vi "SetPosition.vi"(7 "AltPipe?":bool, 8 "error in (no error)":errorcluster, 9 "Position":T1=enum."C0, Cargo Ground", 10 "Hatch Grabbed?":bool, 11 "Elevator Concrete in":refnum<class "Elevator Linear.lvclass">) -> (0 "error out":errorcluster, 3 "Elevator Concrete out":refnum<class "Elevator Linear.lvclass">)   [LabVIEW 2018, in "Elevator.lvlib" / "Elevator Linear.lvclass"]
uses:
  Elevator Linear.lvclass
  C:/Users/Public/Documents/2019DeepSpace/Classes/Elevator/Elevator.lvclass
  Controls/Elevator Position.ctl
  Elevator Linear.lvclass/Elevator Linear.ctl
  Elevator.lvclass/Elevator.ctl
  Public Methods/Read Arm Position Values.vi
  <vilib>/Rock Robotics/Network Tables/NT Write Number.vi
  <vilib>/Rock Robotics/Network Tables/NT Write String.vi
  Elevator.lvclass
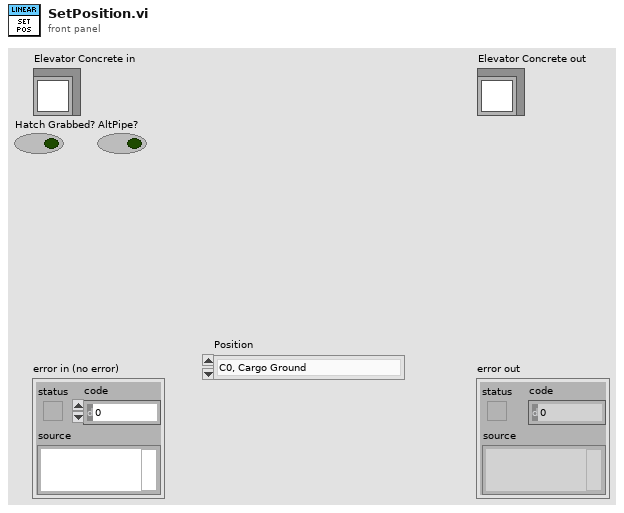
[diagram p1: front panel]
types:
  T1 = typedef "Elevator.lvlib/Elevator.lvclass/Elevator Position.ctl" = enum16{"CS, Cargo Ship Cargo", "C0, Cargo Ground", "C1, LV1 Cargo", "C2, LV2 Cargo", "C3, LV3 Cargo", "H0, LV1 Hatch", "H1, LV2 Hatch", "H2, LV3 Hatch"}
  T2 = typedef "Elevator.lvlib/Elevator.lvclass/Elevator Constants.ctl" = cluster{"Arm Motion Magic Max Velocity":u32, "Arm Motion Magic Max Acceleration":u32, "Wrist Motion Magic Max Velocity":u32, "Wrist Motion Magic Max Acceleration":u32, "Elevator Linear Motion Magic Max Velocity":u32, "Elevator Linear Motion Magic Max Acceleration":u32, "Arm Gear Ratio":dbl, "Wrist Gear Ratio":dbl, "Elevator Linear Gear Ratio":dbl, "Arm Encoder ABS Value":i32, "Wrist Encoder ABS Value":i32}
  T3 = typedef "Elevator.lvlib/Elevator.lvclass/Arm Position Values.ctl" = cluster{"C0 Arm":dbl, "C1 Arm":dbl, "C2 Arm":dbl, "H1 Arm":dbl, "H2 Arm":dbl, "C0 Wrist":dbl, "C1 Wrist ":dbl, "C2 Wrist":dbl, "H1 Wrist":dbl, "H2 Wrist":dbl, "Deploy Arm":dbl, "Deploy Wrist":dbl, "Climb Arm":dbl, "Climb Wrist":dbl, "Stowed Arm":dbl, "Stowed Wrist":dbl, "CS":dbl, "C0":dbl, "C1":dbl, "C2":dbl, "C3":dbl, "H0":dbl, "H1":dbl, "H2":dbl}
  T4 = typedef "WPI_MotorControlDeviceRef.ctl" = cluster{"DeviceStatus":errorcluster, "Type":T5, "PWM":cluster{"PWM Channel":T6, "DeadBand":T7}, "CAN":cluster{"Device Number":u8, "SetOutput VI Ref":variant, "GetOutput VI Ref":variant, "Enable VI Ref":variant, "Disable VI Ref":variant, "Data":variant}, "Invert":bool, "DIO PWM":cluster{"PWM \"Enable\" Channel":T6, "DIOChannel":T8, "PWM Rate":dbl}}
  T5 = typedef "WPI_MotorControlType.ctl" = enum16{"PWM", "CAN", "DIO PWM"}
  T6 = typedef "FPGA_DIOPWMChannel.ctl" = enum8{"PWM 0", "PWM 1", "PWM 2", "PWM 3", "PWM 4", "PWM 5", "PWM 6", "PWM 7", "PWM 8", "PWM 9", "PWM MXP 0", "PWM MXP 1", "PWM MXP 2", "PWM MXP 3", "PWM MXP 4", "PWM MXP 5", "PWM MXP 6", "PWM MXP 7", "PWM MXP 8", "PWM MXP 9", "Invalid"}
  T7 = typedef "WPI_PWMDeadband.ctl" = cluster{"Name":string, "maxPositivePwm":i32, "minPositivePwm":i32, "centerPwm":i32, "maxNegativePwm":i32, "minNegativePwm":i32, "angularRange":u16}
  T8 = typedef "FPGA_DIOChannel.ctl" = enum8{"DIO 0", "DIO 1", "DIO 2", "DIO 3", "DIO 4", "DIO 5", "DIO 6", "DIO 7", "DIO 8", "DIO 9", "DIO MXP 0", "DIO MXP 1", "DIO MXP 2", "DIO MXP 3", "DIO MXP 4", "DIO MXP 5", "DIO MXP 6", "DIO MXP 7", "DIO MXP 8", "DIO MXP 9", "DIO MXP 10", "DIO MXP 11", "DIO MXP 12", "DIO MXP 13", "DIO MXP 14", "DIO MXP 15", "SPI Port CS1", "SPI Port CS2", "SPI Port CS3", "SPI Port MISO", "SPI Port MOSI", "Invalid"}
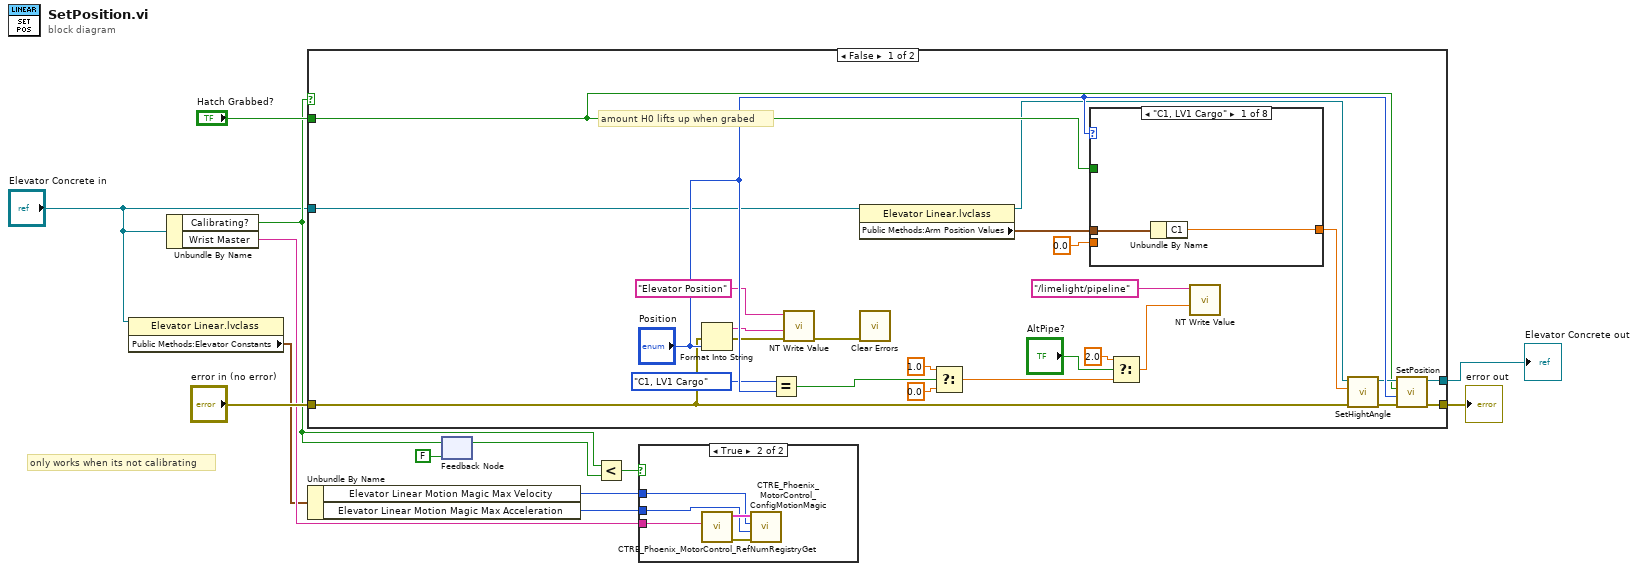
[diagram p0: block diagram]
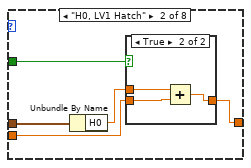
[diagram p3: hidden frame]
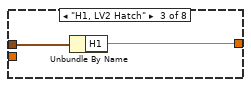
[diagram p5: hidden frame]
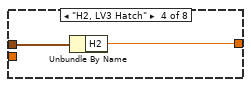
[diagram p6: hidden frame]
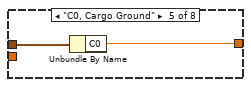
[diagram p7: hidden frame]
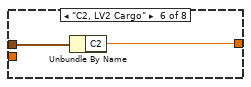
[diagram p8: hidden frame]
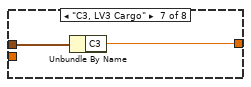
[diagram p9: hidden frame]
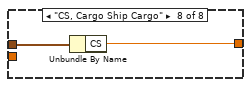
[diagram p10: hidden frame]
diagram:
  # "only works when its not calibrating"
  n1 = property class="Elevator Linear.lvclass"(reference="Elevator Concrete in") -> ("Public Methods:Elevator Constants"=w4:T2)  [unwired: 1 in, 2 out]
  n2 = Unbundle By Name("Elevator Concrete in") -> ("Calibrating?"=w7:bool, "Wrist Master"=w6:string)
  n3 = case shown="False" w7 {
    tunnel: "error in (no error)" -> [w14 w62]
    tunnel: "Elevator Concrete in" -> [w37 w63]
    tunnel: [w36 w62] -> w12
    tunnel: [w35 w63] -> w11
    tunnel: "Hatch Grabbed?" -> [w32 _]
    frame False {
      # "amount H0 lifts up when grabed"
      n4 = Format Into String(error in=w14, "Position") -> (resulting string=w26:string, error out=w27:errorcluster)  [unwired: 2 in]
      n5 = Equal?(x=Elevator_Position."C1, LV1 Cargo" ("Position 2"), y="Position") -> (x = y?=w25:bool)
      n6 = call-poly <vilib>:"NT Write Value.vi"("error in"=w27, "String"=w26, "Name"="Elevator Position") -> ("error out"=w29:errorcluster)  [unwired: 8 in]
      n7 = property class="Elevator Linear.lvclass"(reference=w37) -> (reference out=w31:refnum<class "Elevator Linear.lvclass">, "Public Methods:Arm Position Values"=w17:T3)  [unwired: 1 in, 1 out]
      n8 = call <vilib>:"Clear Errors.vi"("error in (no error)"=w29) -> ()  [unwired: 5 in, 2 out]
      n9 = Select(t=1.0, s=w25, f=0.0) -> (s? t:f=w21:dbl)
      n10 = case shown="\"C1, LV1 Cargo\"" "Position" {
        tunnel: [w39 w43 w50 w52 w54 w56 w58 w60] -> w15
        tunnel: 0.0 -> [_ w44 _ _ _ _ _ _]
        tunnel: w32 -> [_ w45 _ _ _ _ _ _]
        tunnel: w17 -> [w40 w42 w51 w53 w55 w57 w59 w61]
        frame "C1, LV1 Cargo" {
          n11 = Unbundle By Name(w40) -> ("C1"=w39:dbl)
        }
        frame "H0, LV1 Hatch" {
          n12 = Unbundle By Name(w42) -> ("H0"=w41:dbl)
          n13 = case shown="True" w45 {
            tunnel: [w46 w48] -> w43
            tunnel: w44 -> [w46 w49]
            tunnel: w41 -> [_ w47]
            frame False {
            }
            frame True {
              n14 = Add(x=w47, y=w49) -> (x+y=w48:dbl)
            }
          }
        }
        frame "H1, LV2 Hatch" {
          n15 = Unbundle By Name(w51) -> ("H1"=w50:dbl)
        }
        frame "H2, LV3 Hatch" {
          n16 = Unbundle By Name(w53) -> ("H2"=w52:dbl)
        }
        frame "C0, Cargo Ground" {
          n17 = Unbundle By Name(w55) -> ("C0"=w54:dbl)
        }
        frame "C2, LV2 Cargo" {
          n18 = Unbundle By Name(w57) -> ("C2"=w56:dbl)
        }
        frame "C3, LV3 Cargo" {
          n19 = Unbundle By Name(w59) -> ("C3"=w58:dbl)
        }
        frame "CS, Cargo Ship Cargo" {
          n20 = Unbundle By Name(w61) -> ("CS"=w60:dbl)
        }
      }
      n21 = Select(t=2.0, s="AltPipe?", f=w21) -> (s? t:f=w20:dbl)
      n22 = call-poly <vilib>:"NT Write Value.vi"("Numeric"=w20, "Name"="/limelight/pipeline") -> ()  [unwired: 9 in, 1 out]
      n23 = call-dynamic "SetHightAngle.vi"("error in (no error)"=w14, "Main Input"=w15, "Elevator Concrete in"=w31) -> ("error out"=w34:errorcluster, "Elevator Concrete out"=w33:refnum<class "Elevator Linear.lvclass">)  [unwired: 7 in]
      n24 = call-parent "SetPosition.vi"("error in (no error)"=w34, "Position"="Position", "Hatch Grabbed?"=w32, "Elevator in"=w33) -> ("error out"=w36:errorcluster, "Elevator out"=w35:refnum<class "Elevator Linear.lvclass">)  [unwired: 6 in]
    }
    frame True {
      # "If the elevator is calibrating it will recieve no other input until it is complete"
    }
  }
  "error out" <- w12
  "Elevator Concrete out" <- w11
  n25 = Unbundle By Name(w4) -> ("Elevator Linear Motion Magic Max Velocity"=w3:u32, "Elevator Linear Motion Magic Max Acceleration"=w2:u32)
  n26 = feedback #1(FALSE ("Calibrating?")) -> (w8:bool)
  n27 = feedback-in #1(w7) -> ()
  n28 = Less?(x=w7, y=w8) -> (x < y?=w1:bool)
  n29 = case shown="True" w1 {
    tunnel: w6 -> [_ w68]
    tunnel: w3 -> [_ w65]
    tunnel: w2 -> [_ w64]
    frame False {
    }
    frame True {
      n30 = call <vilib>:"CTRE_Phoenix_MotorControl_RefNumRegistryGet.vi"("refnum name"=w68) -> ("error out"=w67:errorcluster, "PhoenixMotorControlDevRef"=w66:T4)  [unwired: 9 in]
      n31 = call <vilib>:"CTRE_Phoenix_MotorControl_ConfigMotionMagic.vi"("error in (no error)"=w67, "Acceleration"=w64, "Cruise Velocity"=w65, "PhoenixMotorControlDevRef"=w66) -> ()  [unwired: 6 in, 2 out]
    }
  }
